vi "File_logfile.vi"(7 "Command":T1, 8 "error in (no error)":errorcluster, 11 "Comments":string) -> (0 "error out":errorcluster, 2 "selected path":path)   [LabVIEW 2017]
uses:
  File_Module Control.ctl
panel:
  out "date/time string":string
  out "String":string="C:\\Users\\usuario\\Documents\\LabVIEW Data\\logUnique\\"
  out "Fichero_actual":path
  out "Old day":i32
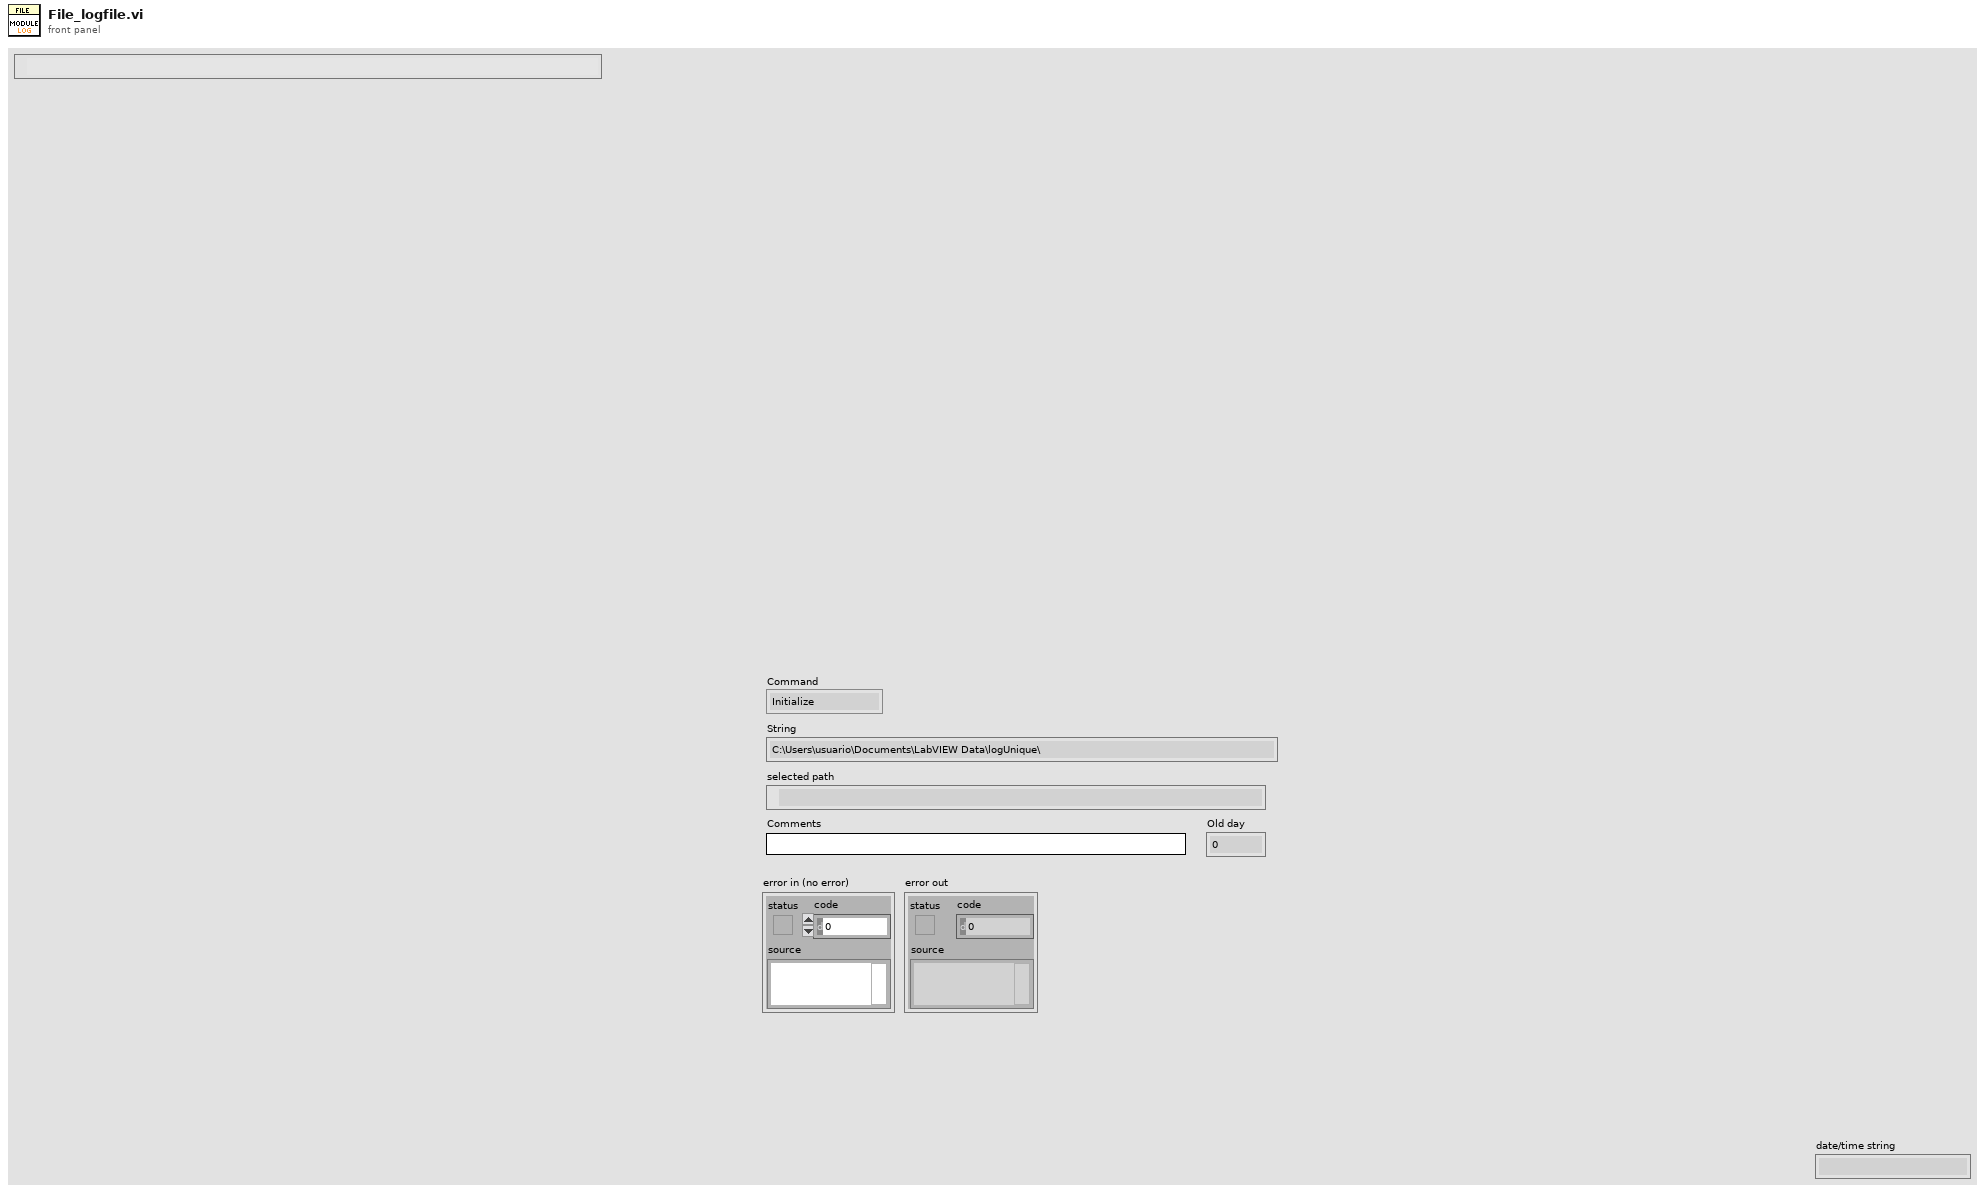
[diagram p1: front panel]
types:
  T1 = typedef "File_Module Control.ctl" = enum16{"Initialize", "Save Head", "Save Data", "Shutdown"}
  T2 = enum16{"open", "replace", "create", "open or create", "replace or create", "replace or create with confirmation"}
  T3 = typedef "LVDateTimeRec.ctl" = cluster{"fractional second":dbl, "second":i32, "minute":i32, "hour":i32, "day of month":i32, "month":i32, "year":i32, "day of week":i32, "day of year":i32, "DST":i32}
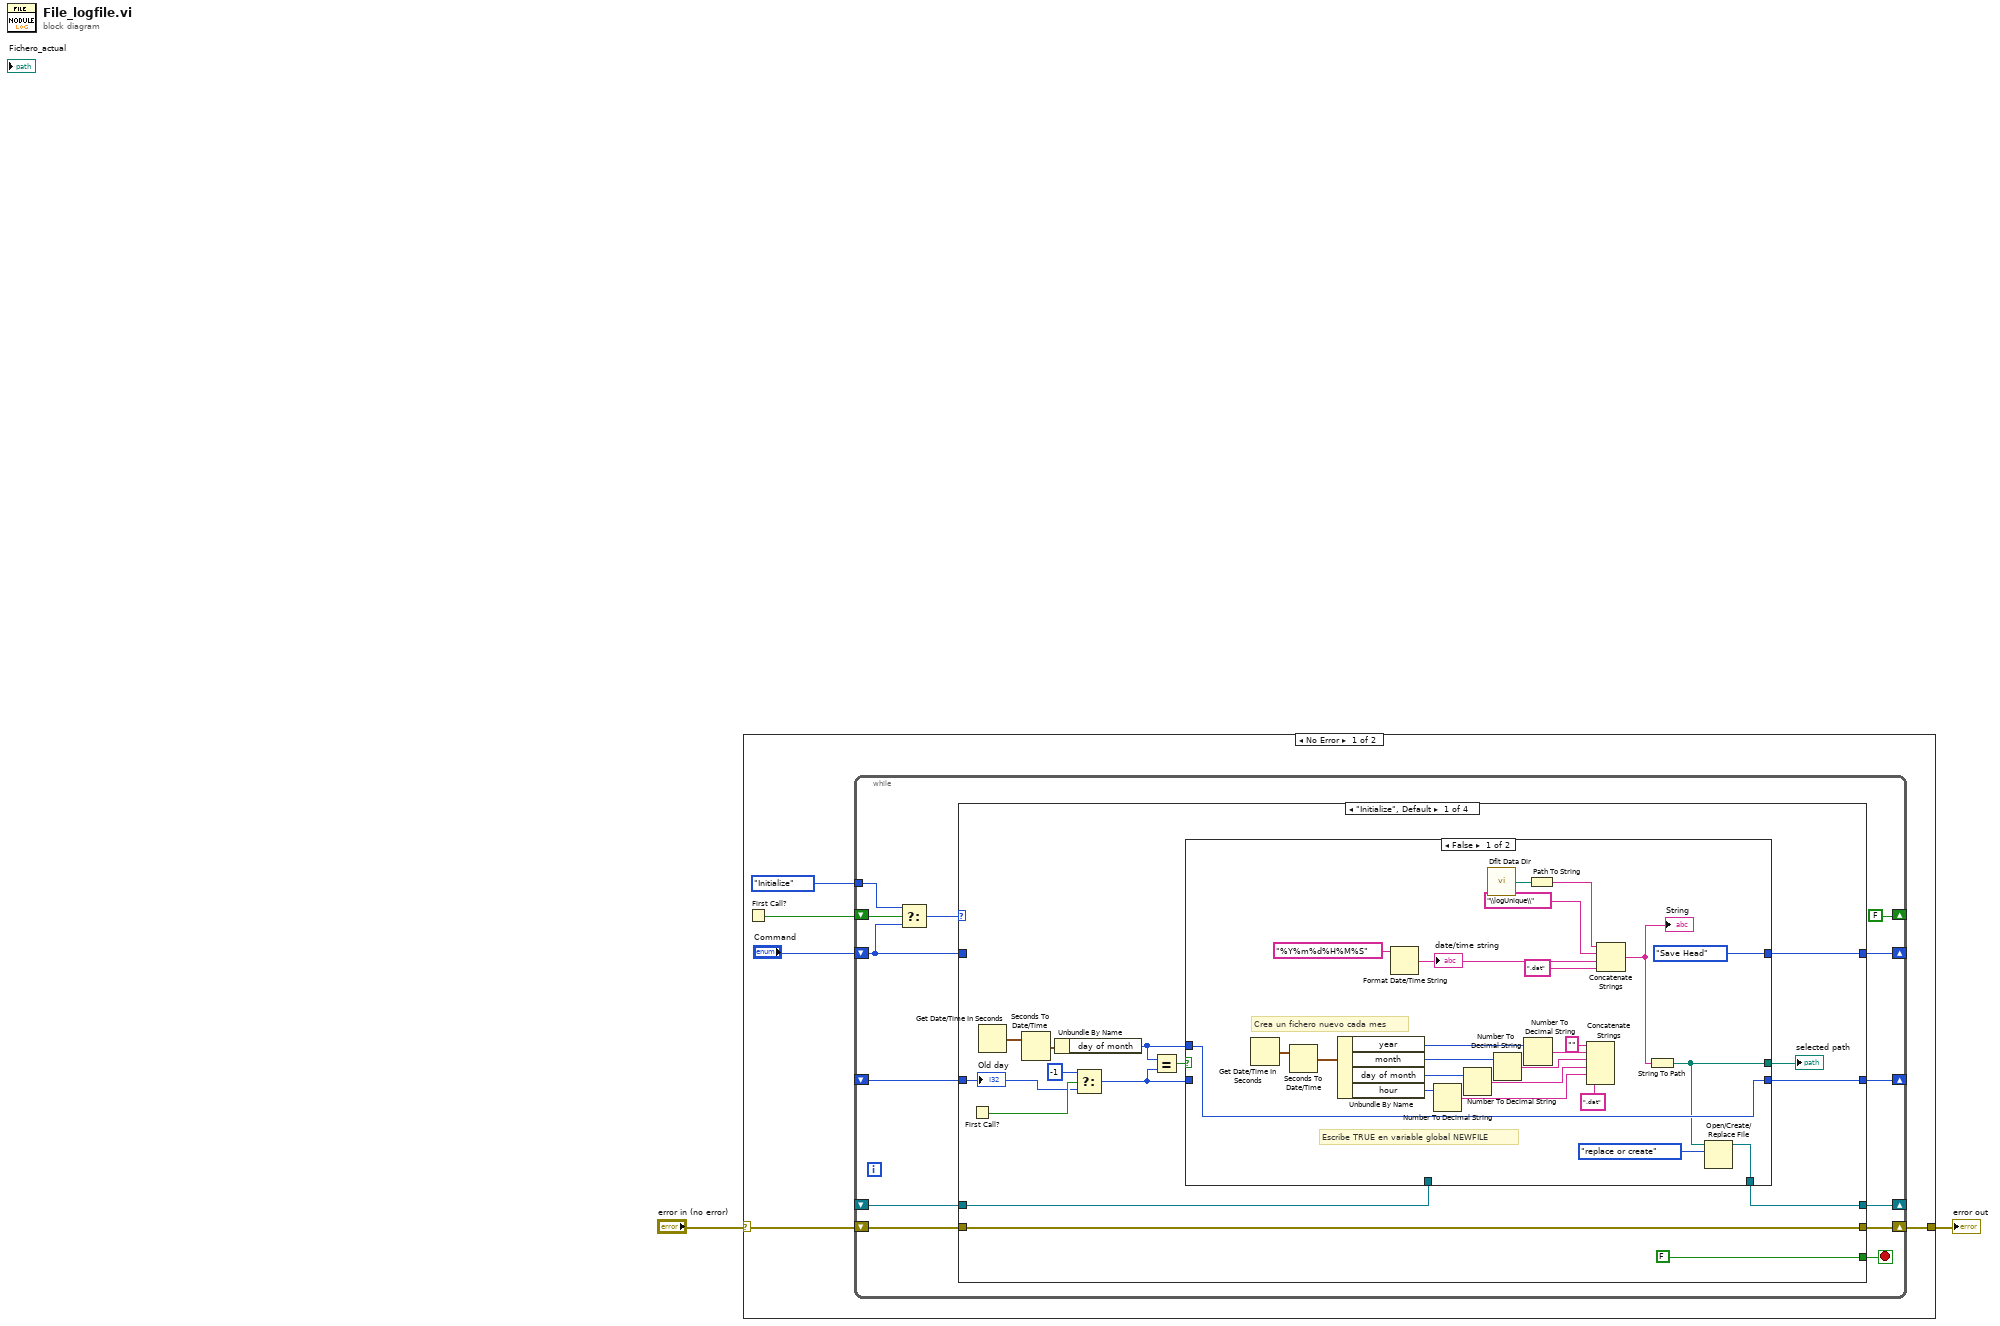
[diagram p0: block diagram]
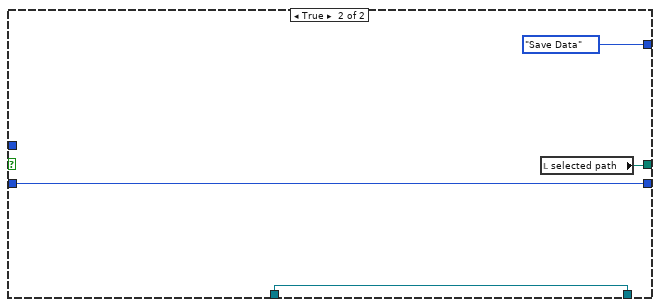
[diagram p2: hidden frame]
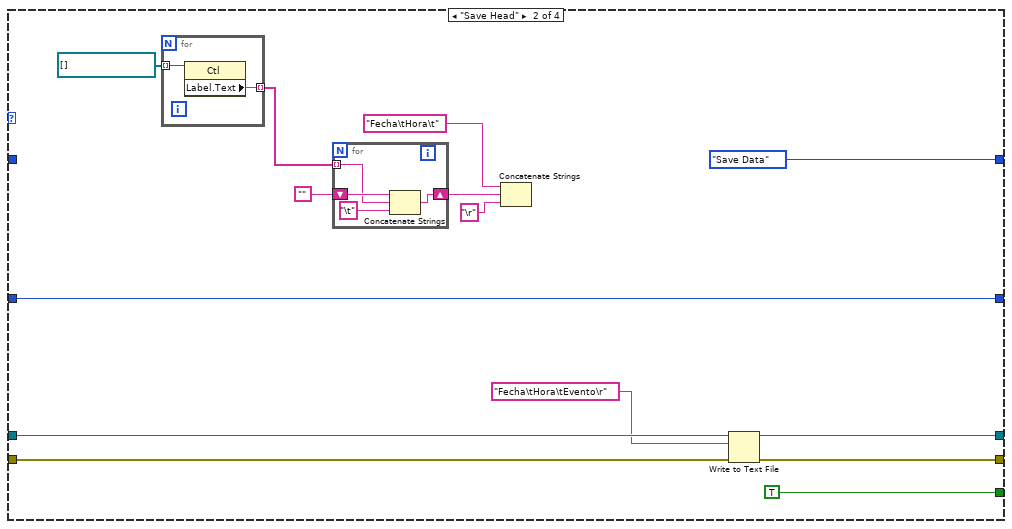
[diagram p3: hidden frame]
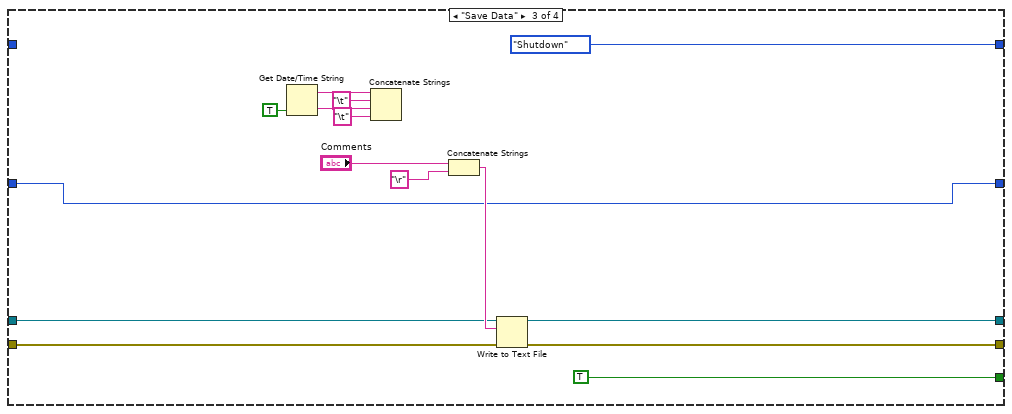
[diagram p4: hidden frame]
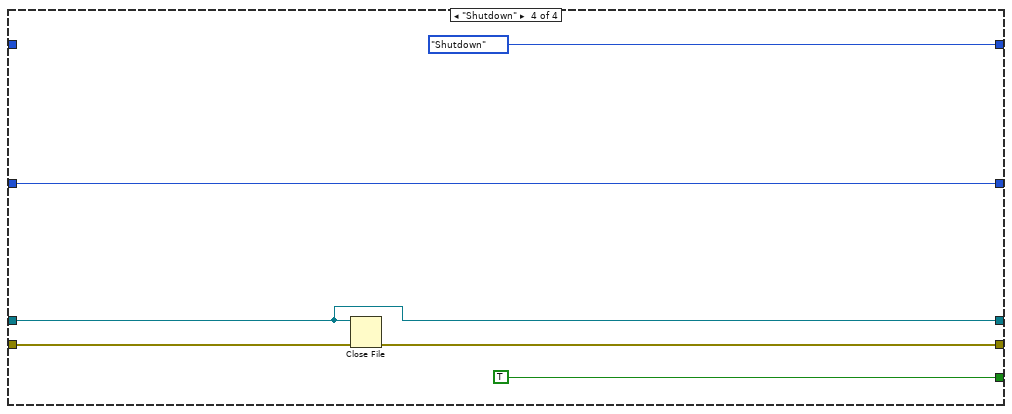
[diagram p5: hidden frame]
diagram:
  n1 = case shown="No Error" "error in (no error)" {
    selector: "error in (no error)" -> [w5 w105]
    tunnel: [w4 w105] -> w1
    frame No Error {
      n2 = First Call?() -> (First Call?: T/F=w7:bool)
      n3 = while {
        shift-right: [w12] -> _
        shift-left: "Command" -> [w13]
        shift-right: [w15] -> w4
        shift-left: w5 -> [w16]
        shift-right: [FALSE ("First Call?: T/F")] -> _
        shift-left: w7 -> [w20]
        tunnel: File_Module_Control."Initialize" ("t") -> [w19]
        shift-right: [w10] -> _
        shift-left: _ -> [w11]
        shift-right: [w8] -> _
        shift-left: _ -> [w9]
        stop <- w17 stop-if-true
        n4 = Select(t=w19, s=w20, f=w13) -> (s? t:f=w18:T1)
        n5 = case shown="\"Initialize\", Default" w18 {
          tunnel: [FALSE TRUE TRUE TRUE] -> w17
          tunnel: w16 -> [w29 w73 w96 w102]
          tunnel: [w29 w72 w95 w101] -> w15
          tunnel: w13 -> [_ _ _ _]
          tunnel: [w27 File_Module_Control."Save Data" ("t") File_Module_Control."Shutdown" File_Module_Control."Shutdown"] -> w12
          tunnel: w11 -> [w28 w75 w92 w100]
          tunnel: [w30 w74 w94 w100] -> w10
          tunnel: w9 -> [w23 w67 w86 w99]
          tunnel: [w26 w67 w86 w99] -> w8
          frame "Initialize", Default {
            n6 = First Call?() -> (First Call?: T/F=w25:bool)
            n7 = Get Date/Time In Seconds() -> (seconds since 1Jan1904=w33:timestamp)
            n8 = Seconds To Date/Time(time stamp (now)=w33) -> (date time rec=w34:T3)  [unwired: 1 in]
            n9 = Unbundle By Name(w34) -> ("day of month"=w32:i32)
            n10 = Select(t=-1, s=w25, f=w23) -> (s? t:f=w22:i32)
            n11 = Equal?(x=w32, y=w22) -> (x = y?=w31:bool)
            n12 = case shown="False" w31 {
              tunnel: w32 -> [w45 _]
              tunnel: w22 -> [_ w61]
              tunnel: [w47 w63] -> w30
              tunnel: w28 -> [_ w63]
              tunnel: [File_Module_Control."Save Head" ("t") File_Module_Control."Save Data" ("t")] -> w27
              tunnel: [w45 w61] -> w26
              tunnel: [w44 w60] -> w21
              frame False {
                # "Escribe TRUE en variable global NEWFILE"
                # "Crea un fichero nuevo cada mes"
                n13 = Get Date/Time In Seconds() -> (seconds since 1Jan1904=w52:timestamp)
                n14 = Seconds To Date/Time(time stamp (now)=w52) -> (date time rec=w53:T3)  [unwired: 1 in]
                n15 = Unbundle By Name(w53) -> ("year"=w51:i32, "month"=w49:i32, "day of month"=w55:i32, "hour"=w56:i32)
                n16 = Format Date/Time String(time format string (%c)="%Y%m%d%H%M%S") -> (date/time string=w42:string)  [unwired: 2 in]
                "date/time string" <- w42
                n17 = Number To Decimal String(number=w56) -> (decimal integer string=w58:string)  [unwired: 1 in]
                n18 = Number To Decimal String(number=w55) -> (decimal integer string=w57:string)  [unwired: 1 in]
                n19 = call <vilib>:"Dflt Data Dir.vi"() -> ("App:Default Data Directory"=w40:path)
                n20 = Number To Decimal String(number=w49) -> (decimal integer string=w54:string)  [unwired: 1 in]
                n21 = Number To Decimal String(number=w51) -> (decimal integer string=w50:string)  [unwired: 1 in]
                n22 = Path To String(path=w40) -> (string=w39:string)
                n23 = Concatenate Strings("" ("string"), w50, w54, w57, w58, ".dat") -> ()  [unwired: 1 out]
                n24 = Concatenate Strings(w39, "\\logUnique\\" ("time format string (%c)"), w42, ".dat") -> (w37:string)
                "String" <- w37
                n25 = String To Path(string=w37) -> (path=w44:path)
                n26 = Open/Create/Replace File(file path (use dialog)=w44, operation (0:open)=T2."replace or create") -> (refnum out=w47:refnum<file>)  [unwired: 4 in, 2 out]
              }
              frame True {
                n27 = local read "selected path"() -> (w60:path)
              }
            }
            "selected path" <- w21
            "Old day" <- w23
          }
          frame "Save Head" {
            n28 = for {
              tunnel: refnum<vi>[] [] ("Controls[]") -> [w83] mode=indexing
              tunnel: [w82] -> w68 mode=indexing
              n29 = property class="Ctl"(reference=w83) -> ("Label.Text"=w82:string)  [unwired: 1 in, 2 out]
            }
            n30 = for {
              tunnel: w68 -> [w80] mode=indexing
              shift-right: [w79] -> w71
              shift-left: "" -> [w81]
              n31 = Concatenate Strings(w81, w80, "\t" ("string")) -> (w79:string)
            }
            n32 = Concatenate Strings("Fecha\tHora\t" ("string"), w71, "\r" ("string")) -> ()  [unwired: 1 out]
            n33 = Write to Text File(file (use dialog)=w75, text="Fecha\tHora\tEvento\r" ("string"), error in=w73) -> (refnum out=w74:refnum<file>, error out=w72:errorcluster)  [unwired: 1 in, 1 out]
          }
          frame "Save Data" {
            n34 = Get Date/Time String(want seconds? (F)=TRUE) -> (date string=w89:string, time string=w88:string)  [unwired: 2 in]
            n35 = Concatenate Strings(w89, "\t" ("string"), w88, "\t" ("string")) -> ()  [unwired: 1 out]
            n36 = Concatenate Strings("Comments", "\r" ("string")) -> (w93:string)
            n37 = Write to Text File(file (use dialog)=w92, text=w93, error in=w96) -> (refnum out=w94:refnum<file>, error out=w95:errorcluster)  [unwired: 1 in, 1 out]
          }
          frame "Shutdown" {
            n38 = Close File(refnum=w100, error in=w102) -> (error out=w101:errorcluster)  [unwired: 1 out]
          }
        }
      }
    }
    frame Error {
    }
  }
  "error out" <- w1
